vi "Rename.vi"() -> ()   [LabVIEW 2025]
uses:
  _Rename/_Rename/_Rename.lvclass
  _Shared/_Shared.lvlib
  _Shared/Tree/Tree.lvlib
  _Shared/Panel/Panel.lvlib
  _Shared/Name Specs/Name Specs.lvclass
panel:
  out "Target":string
  in  "Tree":string(tree)
  in  "OK":bool
  in  "Rename":string
  # "Disclaimer: Please consider committing changes before AND after this action"
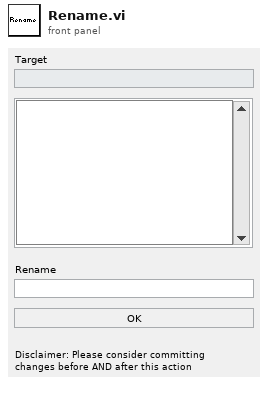
[diagram p1: front panel]
types:
  T1 = typedef "_Shared.lvlib/Type Name Library File Path.ctl" = map{T2, T3}
  T2 = typedef "_Shared.lvlib/Type.ctl" = enum16{"Actor", "Msg"}
  T3 = typedef "_Shared.lvlib/Name Library File Path.ctl" = map{string, path}
  T4 = typedef "_Shared.lvlib/Name Stuff.ctl" = cluster{"Type (Enum)":T2, "Type (String)":string, "Name Library File Path":path, "Name":string, "Name Type":string}
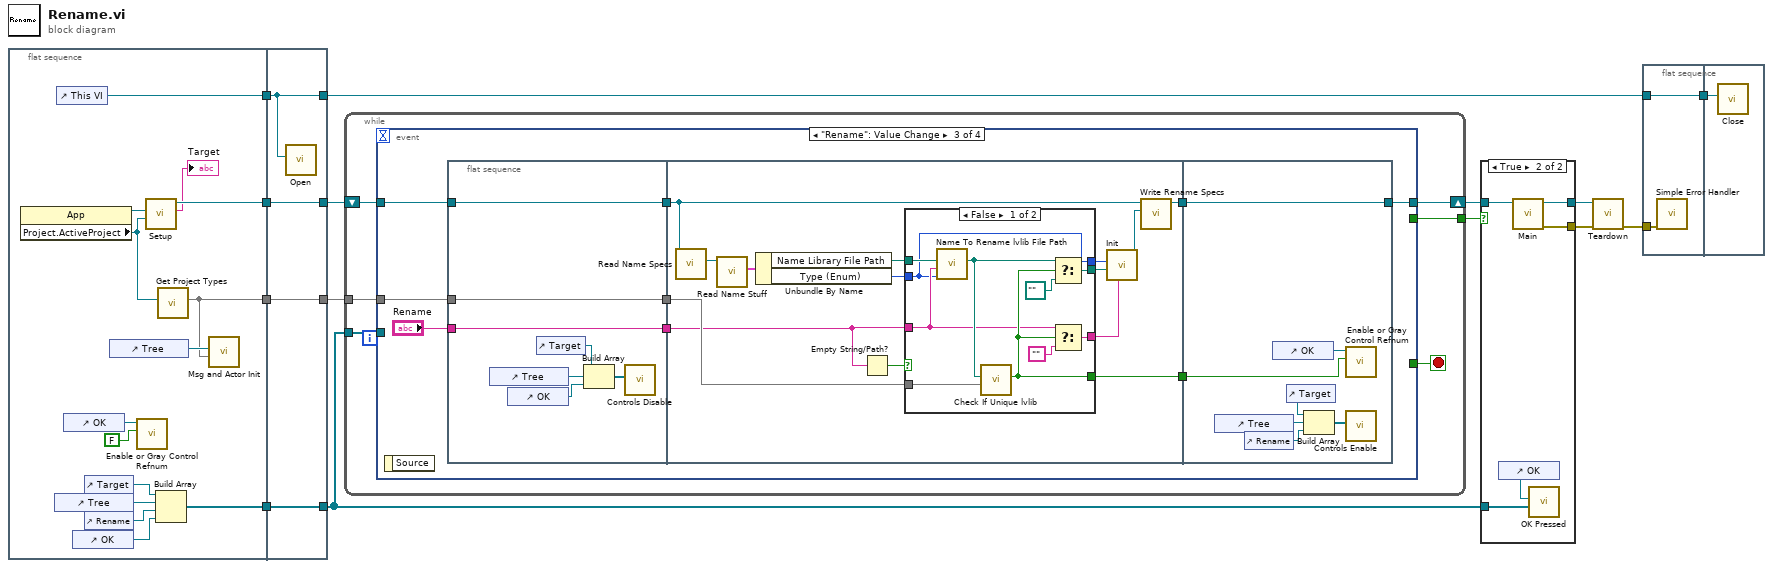
[diagram p0: block diagram]
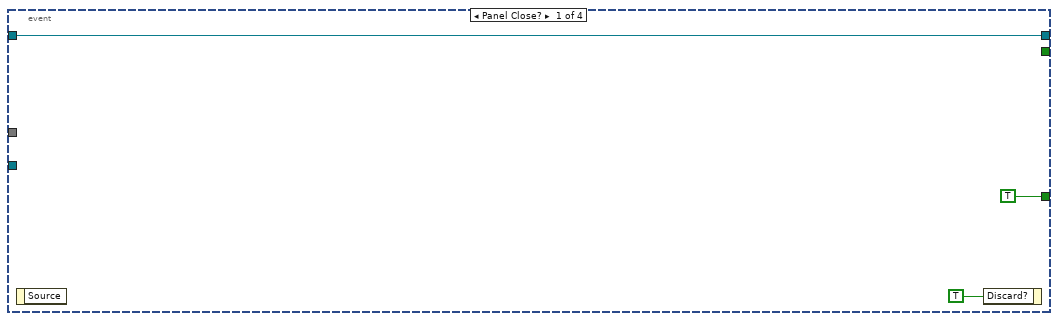
[diagram p2: hidden frame]
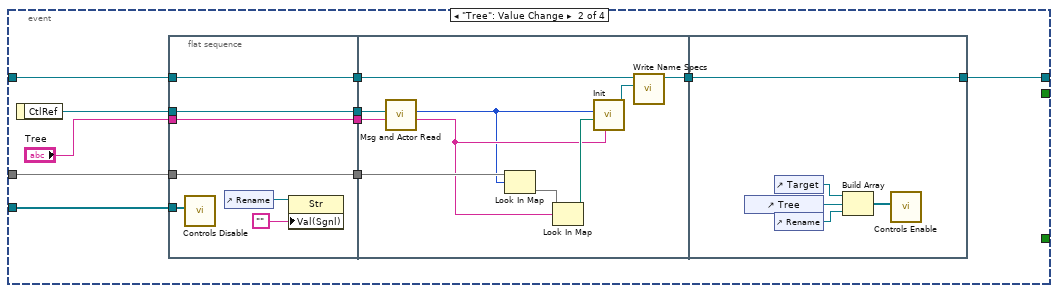
[diagram p3: hidden frame]
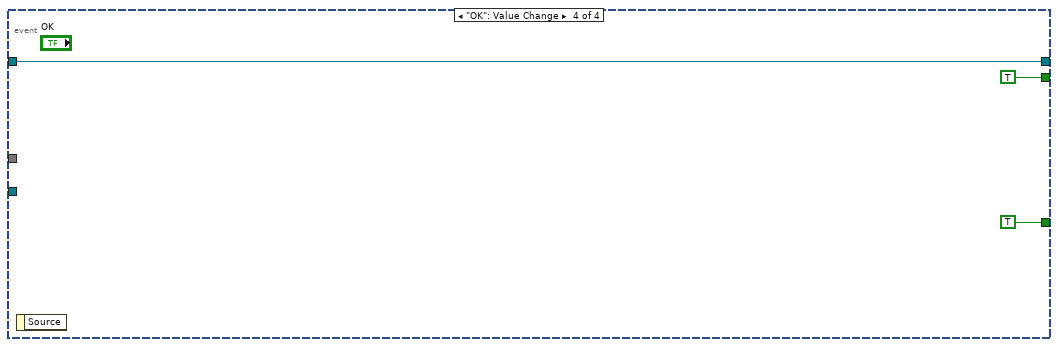
[diagram p5: hidden frame]
diagram:
  n1 = flat-sequence {
    tunnel: [w25] -> w9
    tunnel: [w24] -> w7
    tunnel: [w20] -> w6
    tunnel: [w19] -> w4
    tunnel: [w32] -> w10
    tunnel: w9 -> [w32]
    tunnel: [w31] -> w8
    tunnel: w7 -> [w31]
    tunnel: [w30] -> w5
    tunnel: w6 -> [w30]
    tunnel: w4 -> [w29]
    tunnel: [w29] -> w3
    frame #0 {
      n2 = property class="App"() -> (reference out=w26:refnum<vi>, "Project.ActiveProject"=w27:refnum<vi>)  [unwired: 2 in, 1 out]
      n3 = control-ref of="Tree"() -> (w23:refnum<vi>)
      n4 = control-ref of="This VI"() -> (w19:refnum<vi>)
      n5 = control-ref of="OK"() -> (w18:refnum<vi>)
      n6 = control-ref of="OK"() -> (w21:refnum<vi>)
      n7 = control-ref of="Target"() -> (w15:refnum<vi>)
      n8 = control-ref of="Rename"() -> (w22:refnum<vi>)
      n9 = control-ref of="Tree"() -> (w28:refnum<vi>)
      n10 = call <vilib>:"Enable or Gray Control Refnum.vi"("enable?"=FALSE, "Control in"=w18) -> ()  [unwired: 8 in, 2 out]
      n11 = call "Setup.vi"("Active Project"=w27, "NI.LV.Dialog Instance"=w26) -> ("Target"=→"Target":string, "Script out"=w24:refnum<class "_Rename.lvclass">)  [unwired: 8 in]
      n12 = Build Array(w15, w23, w22, w21) -> (w20:refnum<vi>[])
      n13 = call "Get Project Types.vi"("Project:Active Project"=w27) -> ("Type Name Library File Path"=w25:T1)  [unwired: 10 in]
      n14 = call "Msg and Actor Init.vi"("Type Name Library File Path"=w25, "Tree Ref"=w28) -> ()  [unwired: 10 in]
    }
    frame #1 {
      n15 = call "Open.vi"("VI"=w29) -> ()  [unwired: 11 in]
    }
  }
  n16 = while {
    tunnel: [w38] -> w12
    shift-right: [w35] -> w11
    shift-left: w8 -> [w36]
    tunnel: w10 -> [w34]
    tunnel: w5 -> [w33]
    stop <- w37 stop-if-true
    n17 = event shown="[2] \"Rename\": Value Change" {
      selector: _ -> [_ _ _ _]
      dyn-events: _ -> [_ _ _ _]
      timeout: _ -> [_ _ _ _]
      tunnel: [_ _ _ TRUE ("Rename 2")] -> w38
      tunnel: [TRUE _ _ TRUE] -> w37
      tunnel: w36 -> [w39 w50 w80 w122]
      tunnel: [w39 w52 w83 w122] -> w35
      tunnel: w34 -> [_ w49 w79 _]
      tunnel: w33 -> [_ w42 _ _]
      event Panel Close? {
        n18 = event-data() -> ()  [unwired: 1 in, 1 out]
        n19 = event-data("Discard?"=TRUE) -> ()  [unwired: 1 in, 1 out]
      }
      event "Tree": Value Change {
        n20 = event-data() -> ("CtlRef"=w47:refnum<vi>)  [unwired: 1 in]
        n21 = flat-sequence {
          tunnel: w47 -> [w56]
          tunnel: "Tree" -> [w57]
          tunnel: w49 -> [w58]
          tunnel: w50 -> [w59]
          tunnel: [w59] -> w46
          tunnel: [w58] -> w45
          tunnel: [w57] -> w44
          tunnel: [w56] -> w43
          tunnel: w42 -> [w55]
          tunnel: [w61] -> w51
          tunnel: w46 -> [w62]
          tunnel: w45 -> [w68]
          tunnel: w44 -> [w67]
          tunnel: w43 -> [w66]
          tunnel: [w71] -> w52
          tunnel: w51 -> [w71]
          frame #0 {
            n22 = call "Controls Disable.vi"("Controls in"=w55) -> ()  [unwired: 11 in]
            n23 = control-ref of="Rename"() -> (w54:refnum<vi>)
            n24 = property class="Str"(reference=w54, "Val(Sgnl)"="") -> ()  [unwired: 1 in, 2 out]
          }
          frame #1 {
            n25 = call "Msg and Actor Read.vi"("Tree"=w67, "Tree Ref"=w66) -> ("Name"=w63:string, "Type"=w60:T2)  [unwired: 8 in]
            n26 = Look In Map(map=w68, key=w60) -> (value=w69:T3)  [unwired: 1 in, 1 out]
            n27 = Look In Map(map=w69, key=w63) -> (value=w64:path)  [unwired: 1 in, 1 out]
            n28 = call "Init.vi"("Name"=w63, "Name Library File Path"=w64, "Type"=w60) -> ("Name Specs out"=w65:refnum<class "Name Specs.lvclass">)  [unwired: 8 in]
            n29 = call "Write Name Specs.vi"("Name Specs"=w65, "_Rename in"=w62) -> ("_Rename out"=w61:refnum<class "_Rename.lvclass">)  [unwired: 9 in]
          }
          frame #2 {
            n30 = control-ref of="Tree"() -> (w73:refnum<vi>)
            n31 = control-ref of="Target"() -> (w70:refnum<vi>)
            n32 = control-ref of="Rename"() -> (w74:refnum<vi>)
            n33 = Build Array(w70, w73, w74) -> (w72:refnum<vi>[])
            n34 = call "Controls Enable.vi"("Controls in"=w72) -> ()  [unwired: 11 in]
          }
        }
      }
      event "Rename": Value Change {
        n35 = event-data() -> ()  [unwired: 1 in, 1 out]
        n36 = flat-sequence {
          tunnel: "Rename" -> [w88]
          tunnel: w79 -> [w89]
          tunnel: w80 -> [w90]
          tunnel: [w90] -> w77
          tunnel: [w89] -> w76
          tunnel: [w88] -> w75
          tunnel: [w101] -> w82
          tunnel: [w94] -> w81
          tunnel: w77 -> [w93]
          tunnel: w76 -> [w103]
          tunnel: w75 -> [w102]
          tunnel: [w116] -> w83
          tunnel: w82 -> [w117]
          tunnel: w81 -> [w116]
          frame #0 {
            n37 = control-ref of="Tree"() -> (w85:refnum<vi>)
            n38 = control-ref of="OK"() -> (w86:refnum<vi>)
            n39 = control-ref of="Target"() -> (w84:refnum<vi>)
            n40 = Build Array(w84, w85, w86) -> (w87:refnum<vi>[])
            n41 = call "Controls Disable.vi"("Controls in"=w87) -> ()  [unwired: 11 in]
          }
          frame #1 {
            n42 = call "Read Name Specs.vi"("_Rename in"=w93) -> ("Name Specs"=w100:refnum<class "Name Specs.lvclass">)  [unwired: 10 in]
            n43 = call "Read Name Stuff.vi"("Name Specs in"=w100) -> ("Name Stuff"=w99:T4)  [unwired: 10 in]
            n44 = Unbundle By Name(w99) -> ("Name Library File Path"=w98:path, "Type (Enum)"=w92:T2)
            n45 = Empty String/Path?(string/path=w102) -> (empty?=w104:bool)
            n46 = case shown="False" w104 {
              tunnel: [w112 _] -> w101
              tunnel: w103 -> [w107 _]
              tunnel: w102 -> [w106 _]
              tunnel: [w109 _] -> w95
              tunnel: [w114 _] -> w96
              tunnel: w98 -> [w113 _]
              tunnel: w92 -> [w105 _]
              tunnel: [w105 _] -> w91
              frame False {
                n47 = call "Name To Rename lvlib File Path.vi"("Type"=w105, "Rename"=w106, "Name Library File Path"=w113) -> ("Rename Library File Path"=w111:path)  [unwired: 8 in]
                n48 = call "Check If Unique lvlib.vi"("Type Name Library File Path"=w107, "Library File Path"=w111) -> ("Unique?"=w112:bool)  [unwired: 9 in]
                n49 = Select(t=w111, s=w112, f=path "") -> (s? t:f=w109:path)
                n50 = Select(t=w106, s=w112, f="") -> (s? t:f=w114:string)
              }
              frame True {
              }
            }
            n51 = call "Init.vi"("Name"=w96, "Name Library File Path"=w95, "Type"=w91) -> ("Name Specs out"=w97:refnum<class "Name Specs.lvclass">)  [unwired: 8 in]
            n52 = call "Write Rename Specs.vi"("Rename Specs"=w97, "_Rename in"=w93) -> ("_Rename out"=w94:refnum<class "_Rename.lvclass">)  [unwired: 9 in]
          }
          frame #2 {
            n53 = control-ref of="Tree"() -> (w121:refnum<vi>)
            n54 = control-ref of="Rename"() -> (w119:refnum<vi>)
            n55 = control-ref of="OK"() -> (w118:refnum<vi>)
            n56 = control-ref of="Target"() -> (w115:refnum<vi>)
            n57 = Build Array(w115, w121, w119) -> (w120:refnum<vi>[])
            n58 = call <vilib>:"Enable or Gray Control Refnum.vi"("enable?"=w117, "Control in"=w118) -> ()  [unwired: 8 in, 2 out]
            n59 = call "Controls Enable.vi"("Controls in"=w120) -> ()  [unwired: 11 in]
          }
        }
      }
      event "OK": Value Change {
        n60 = event-data() -> ()  [unwired: 1 in, 1 out]
      }
    }
  }
  n61 = case shown="True" w12 {
    tunnel: w11 -> [w125 w130]
    tunnel: [w125 w129] -> w14
    tunnel: w5 -> [_ w126]
    tunnel: [_ w128] -> w13
    frame False {
    }
    frame True {
      n62 = control-ref of="OK"() -> (w127:refnum<vi>)
      n63 = call "Main.vi"("_Rename in"=w130) -> ("error out"=w128:errorcluster, "_Rename out"=w129:refnum<class "_Rename.lvclass">)  [unwired: 9 in]
      n64 = call "OK Pressed.vi"("Controls in"=w126, "OK Ref"=w127) -> ()  [unwired: 10 in]
    }
  }
  n65 = call "Teardown.vi"("error in"=w13, "_Rename in"=w14) -> ("error out"=w1:errorcluster)  [unwired: 9 in]
  n66 = flat-sequence {
    tunnel: w3 -> [w132]
    tunnel: [w132] -> w2
    tunnel: w1 -> [w131]
    tunnel: w2 -> [w133]
    frame #0 {
      n67 = call <vilib>:"Simple Error Handler.vi"("error in (no error)"=w131) -> ()  [unwired: 4 in, 5 out]
    }
    frame #1 {
      n68 = call "Close.vi"("VI"=w133) -> ()  [unwired: 11 in]
    }
  }
